vi "New XWPF Reader.vi"(8 "error in (no error)":errorcluster, 11 "XWPF File Path":path) -> (0 "error out":errorcluster, 3 "xwpfReader out":refnum<class "xwpfReader.lvclass">)   [LabVIEW 2017, in "xwpfReader.lvclass"]
doc: "Opens a FileStream as an input stream. \nCreates an XWPFDocument object using the input stream."
uses:
  xwpfReader.lvclass
  C:/Users/Neo/Desktop/Dev_Tools_BR/LabVIEW_NPOI/lib/NPOI 2.1.1/NPOI.OOXML.dll
  lib/NPOI 2.1.1/NPOI.OOXML.dll
  xwpfReader.lvclass/xwpfReader.ctl
  Support/File Stream/File Stream.lvlib
  <vilib>/Ekim/LUT/LUT/LUT.lvclass
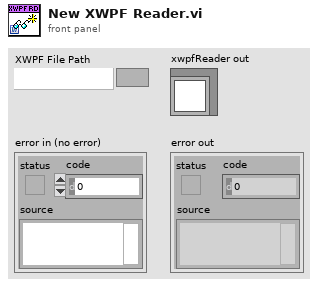
[diagram p1: front panel]
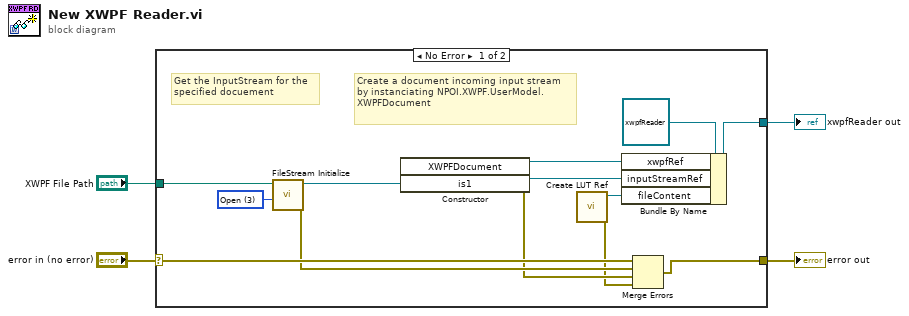
[diagram p0: block diagram]
diagram:
  n1 = case shown="No Error" "error in (no error)" {
    selector: "error in (no error)" -> [w16 w17]
    tunnel: [w15 w17] -> w3
    tunnel: [w13 _] -> w2
    tunnel: "XWPF File Path" -> [w12 _]
    frame No Error {
      w11 = 3 items=["CreateNew"=1, "Create"=2, "Open"=3, "OpenOrCreate"=4, "Truncate"=5, "Append"=6] ("mode")
      # "Create a document incoming input stream by instanciating NPOI.XWPF.UserModel.XWPFDocument"
      # "Get the InputStream for the\nspecified docuement"
      n2 = call "FileStream Initialize.vi"("mode"=w11, "path"=w12) -> ("error out"=w8:errorcluster, "new reference"=w9:refnum<k24>)  [unwired: 8 in]
      n3 = constructor class="XWPFDocument"("is1"=w9) -> (reference out=w10:refnum<k24>, error out=w7:errorcluster)  [unwired: 3 in, 2 out]
      n4 = call <vilib>:"Create LUT Ref.vi"() -> ("error out"=w5:errorcluster, "LUT out"=w6:refnum<class "LUT.lvclass">)  [unwired: 10 in]
      n5 = Bundle By Name(cluster=refnum<class "xwpfReader.lvclass"> refnum ("xwpfReader in"), "xwpfRef"=w10, "inputStreamRef"=w9, "fileContent"=w6) -> (w13:refnum<class "xwpfReader.lvclass">)
      n6 = Merge Errors(w16, w8, w7, w5) -> (w15:errorcluster)
    }
    frame Error {
    }
  }
  "error out" <- w3
  "xwpfReader out" <- w2
